vi "check RTU validity.vi"(7 "RTU transmission data unit in":refnum<class "RTU Data Unit.lvclass">, 8 "error in (no error)":errorcluster, 10 "unit ID":u8, 11 "unsigned byte array":u8[](array[numeric])) -> (0 "error out":errorcluster, 1 "valid packet":bool, 2 "valid PDU":bool, 3 "Modbus Data Unit out":refnum<class "Modbus Data Unit.lvclass">, 5 "RTU transmission data unit out":refnum<class "RTU Data Unit.lvclass">)   [LabVIEW 2013, in "Modbus Library - Advance.lvlib" / "RTU Data Unit.lvclass"]
uses:
  RTU Data Unit.lvclass
  Modbus Data Unit/Modbus Data Unit.lvclass
  Serial Interface/Serial Data Unit.lvclass/Serial Data Unit.ctl
  Modbus Data Unit/Modbus Data Unit.lvclass/Modbus Data Unit.ctl
  Serial Interface/Serial Data Unit.lvclass
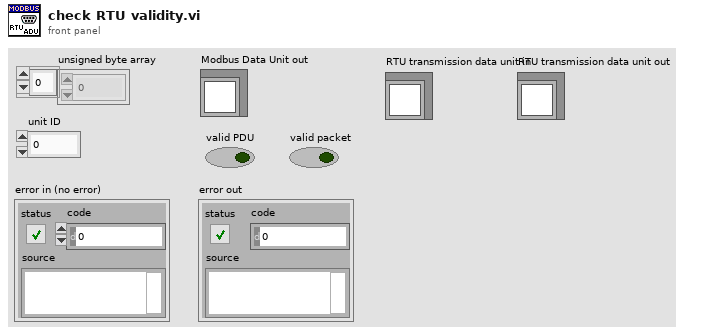
[diagram p1: front panel]
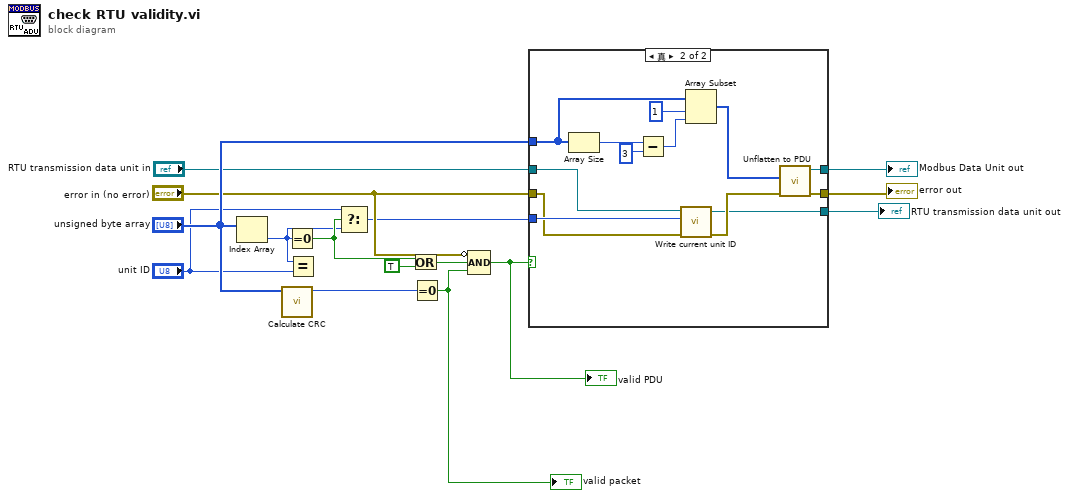
[diagram p0: block diagram]
diagram:
  n1 = Index Array(array="unsigned byte array") -> (element=w5:u8)  [unwired: 1 in]
  n2 = call "Calculate CRC.vi"("data"="unsigned byte array") -> ("CRC-16"=w10:u16)  [unwired: 10 in]
  n3 = Equal To 0?(x=w5) -> (x = 0?=w7:bool)
  n4 = Equal?(x=w5, y="unit ID") -> ()  [unwired: 1 out]
  n5 = Select(t="unit ID", s=w7, f=w5) -> (s? t:f=w3:u8)
  n6 = Or(x=w7, y=TRUE) -> (x .or. y?=w11:bool)
  n7 = Equal To 0?(x=w10) -> (x = 0?=w9:bool)
  "valid packet" <- w9
  n8 = Compound Arithmetic op=AND(invert "error in (no error)", w11, w9) -> (w8:bool)
  "valid PDU" <- w8
  n9 = case shown="真" w8 {
    tunnel: "error in (no error)" -> [w17 w21]
    tunnel: "unsigned byte array" -> [_ w25]
    tunnel: [w17 w24] -> w14
    tunnel: [_ w23] -> w15
    tunnel: w3 -> [_ w22]
    tunnel: "RTU transmission data unit in" -> [w16 w19]
    tunnel: [w16 w18] -> w1
    frame False {
    }
    frame True {
      n10 = Array Size(array=w25) -> (size(s)=w28:i32)
      n11 = Subtract(x=w28, y=3) -> (x-y=w26:i32)
      n12 = call "Write current unit ID.vi"("error in (no error)"=w21, "request unit ID"=w22, "Serial Data Unit in"=w19) -> ("error out"=w20:errorcluster, "Serial Data Unit out"=w18:refnum<class "RTU Data Unit.lvclass">)  [unwired: 7 in]
      n13 = Array Subset(array=w25, index=1, length=w26) -> (w30:u8[])
      n14 = call "Unflatten to PDU.vi"("error in"=w20, "modbus data unit data"=w30) -> ("error out"=w24:errorcluster, "modbus data unit out"=w23:refnum<class "Modbus Data Unit.lvclass">)  [unwired: 8 in]
    }
  }
  "Modbus Data Unit out" <- w15
  "error out" <- w14
  "RTU transmission data unit out" <- w1
